vi "failUnlessEqual.vi"(6 "delta (optional)":variant, 8 "error in (no error)":errorcluster, 9 "y":variant, 10 "x":variant, 11 "TestCase in":refnum<class "TestCase.lvclass">) -> (0 "error out":errorcluster, 3 "TestCase out":refnum<class "TestCase.lvclass">)   [LabVIEW 2011, in "TestCase.lvclass"]
doc: "{Obsolete - kept for compatiblity only}\n\nFail test if 'x' != 'y'. 'delta (optional)' if specified must be a numeric format and forces 'x', 'y' to be numeric. If 'delta' is not specified, x,y can be any variant data."
uses:
  TestCase.lvclass
  Libraries/VITesterUtilities.lvlib
panel:
  # "JKI VI Tester for LabVIEW\nhttp://jkisoft.com/vi-tester\nCopyright (C) 2007-2009, JKI <info@jkisoft.com>\nALL RIGHTS RESERVED"
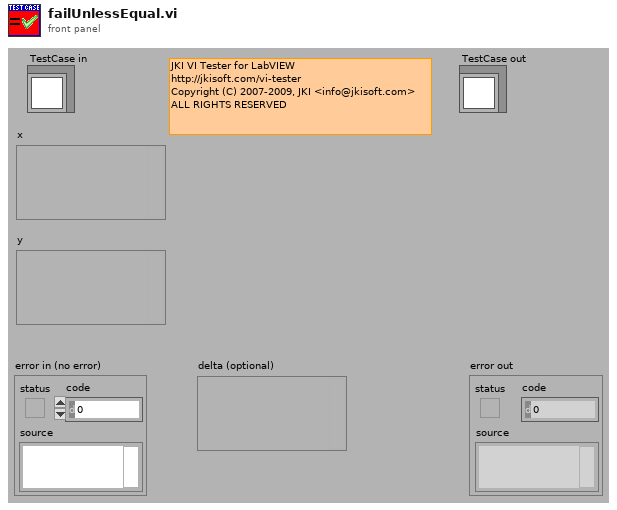
[diagram p1: front panel]
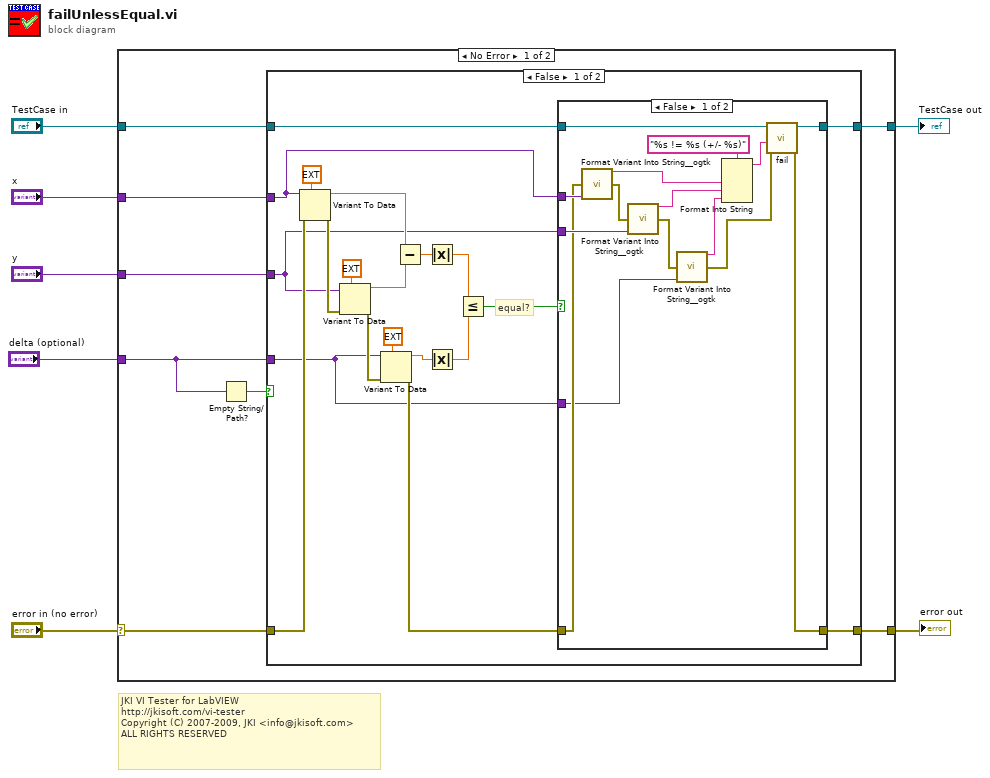
[diagram p0: block diagram]
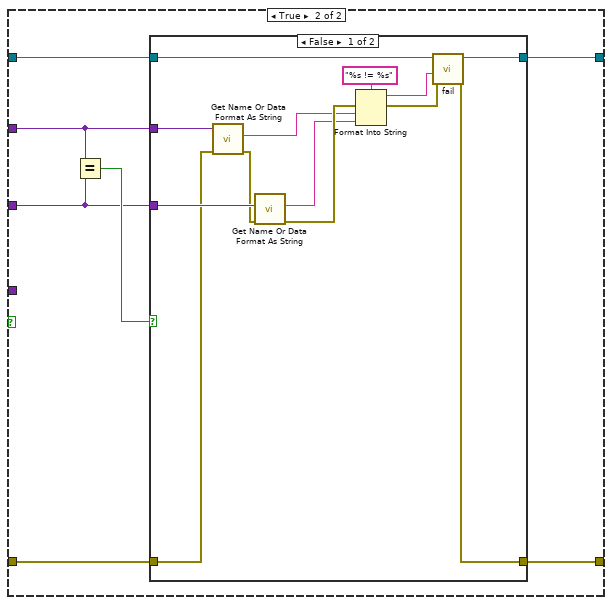
[diagram p3: hidden frame]
diagram:
  # "JKI VI Tester for LabVIEW\nhttp://jkisoft.com/vi-tester\nCopyright (C) 2007-2009, JKI <info@jkisoft.com>\nALL RIGHTS RESERVED"
  n1 = case shown="No Error" "error in (no error)" {
    selector: "error in (no error)" -> [w12 w76]
    tunnel: [w11 w76] -> w6
    tunnel: [w8 w75] -> w4
    tunnel: "TestCase in" -> [w9 w75]
    tunnel: "delta (optional)" -> [w10 _]
    tunnel: "x" -> [w15 _]
    tunnel: "y" -> [w14 _]
    frame No Error {
      n2 = Empty String/Path?(string/path=w10) -> (empty?=w13:bool)
      n3 = case shown="False" w13 {
        tunnel: w15 -> [w18 w54]
        tunnel: w14 -> [w17 w53]
        tunnel: w12 -> [w32 w58]
        tunnel: [w21 w57] -> w11
        tunnel: w10 -> [w16 _]
        tunnel: w9 -> [w20 w56]
        tunnel: [w19 w55] -> w8
        frame False {
          # "equal?"
          n4 = Variant To Data(error in=w32, type=ext 0.0, Variant=w18) -> (data=w29:ext, error out=w33:errorcluster)
          n5 = Variant To Data(error in=w33, type=ext 0.0, Variant=w17) -> (data=w28:ext, error out=w30:errorcluster)
          n6 = Variant To Data(error in=w30, type=ext 0.0, Variant=w16) -> (data=w26:ext, error out=w22:errorcluster)
          n7 = Subtract(x=w29, y=w28) -> (x-y=w27:ext)
          n8 = Absolute Value(x=w27) -> (abs(x)=w25:ext)
          n9 = Absolute Value(x=w26) -> (abs(x)=w24:ext)
          n10 = Less Or Equal?(x=w25, y=w24) -> (x <= y?=w23:bool)
          n11 = case shown="False" w23 {
            tunnel: [w50 w52] -> w21
            tunnel: w22 -> [w44 w52]
            tunnel: w20 -> [w49 w51]
            tunnel: [w48 w51] -> w19
            tunnel: w18 -> [w47 _]
            tunnel: w17 -> [w45 _]
            tunnel: w16 -> [w39 _]
            frame False {
              n12 = call <userlib>:"Format Variant Into String__ogtk.vi"("error in (no error)"=w44, "Variant"=w47) -> ("Output String"=w42:string, "error out"=w46:errorcluster)  [unwired: 12 in]
              n13 = call <userlib>:"Format Variant Into String__ogtk.vi"("error in (no error)"=w46, "Variant"=w45) -> ("Output String"=w43:string, "error out"=w37:errorcluster)  [unwired: 12 in]
              n14 = call <userlib>:"Format Variant Into String__ogtk.vi"("error in (no error)"=w37, "Variant"=w39) -> ("Output String"=w38:string, "error out"=w36:errorcluster)  [unwired: 12 in]
              n15 = Format Into String(format string="%s != %s (+/- %s)", w42, w43, w38) -> (resulting string=w40:string)  [unwired: 2 in, 1 out]
              n16 = call-dynamic "fail.vi"("error in (no error)"=w36, "message (\"\")"=w40, "TestCase in"=w49) -> ("error out"=w50:errorcluster, "TestCase out"=w48:refnum<class "TestCase.lvclass">)  [unwired: 7 in]
            }
            frame True {
            }
          }
        }
        frame True {
          n17 = Equal?(x=w54, y=w53) -> (x = y?=w59:bool)
          n18 = case shown="False" w59 {
            tunnel: w58 -> [w64 w73]
            tunnel: [w70 w73] -> w57
            tunnel: w56 -> [w69 w74]
            tunnel: [w68 w74] -> w55
            tunnel: w54 -> [w66 _]
            tunnel: w53 -> [w65 _]
            frame False {
              n19 = call "Get Name Or Data Format As String.vi"("error in (no error)"=w64, "Data"=w66) -> ("error out"=w63:errorcluster, "Data Value OR Name"=w60:string)  [unwired: 8 in]
              n20 = call "Get Name Or Data Format As String.vi"("error in (no error)"=w63, "Data"=w65) -> ("error out"=w62:errorcluster, "Data Value OR Name"=w61:string)  [unwired: 8 in]
              n21 = Format Into String(format string="%s != %s", error in=w62, w60, w61) -> (resulting string=w71:string, error out=w67:errorcluster)  [unwired: 1 in]
              n22 = call-dynamic "fail.vi"("error in (no error)"=w67, "message (\"\")"=w71, "TestCase in"=w69) -> ("error out"=w70:errorcluster, "TestCase out"=w68:refnum<class "TestCase.lvclass">)  [unwired: 7 in]
            }
            frame True {
            }
          }
        }
      }
    }
    frame Error {
    }
  }
  "error out" <- w6
  "TestCase out" <- w4
